vi "Instrumentation Controls.vi"() -> ()   [LabVIEW 2018]
doc: "This example shows how to use autosetup and acquire a waveform on a single channel."
uses:
  <instrlib>/RIGOL DG4000 Series/Public/Configure/Configure Standard Waveform(Sine).vi
  <instrlib>/RIGOL DS1000 Series/Public/Data/Read (Multiple Waveforms).vi
  <instrlib>/RIGOL DS1000 Series/RIGOL DS1000 Series.lvlib
  <instrlib>/RIGOL DM3058/RIGOL DM3058.lvlib
  <instrlib>/RIGOL DG4000 Series/RIGOL DG4000 Series.lvlib
panel:
  in  "Tab Control":enum32{"DG4062", "DM3068", "DS1204B"}(tab)
  in  "VISA resource name 2":refnum<visa-resource-name>
  in  "Amplitude (0.1 Vpp)":dbl=0.1
  in  "Frequency (1000 Hz)":dbl=1000.0
  in  "DC Offset (0.00 V)":dbl
  in  "Channel":dbl
  in  "Enable Output":bool=TRUE
  in  "VISA resource name 3":refnum<visa-resource-name>
  out "Measurement 3":dbl(knob) scale=0.0..5.0
  in  "Function (0: DC Volts) 2":u16(ring) items=["DC Volts", "AC Volts", "DC Current", "AC Current", "2-Wire Resistance", "4-Wire Resistance"]
  in  "Manual Range (1.0) 2":dbl=1.0
  in  "Auto Range (T: Enable) 2":bool=TRUE
  out "Measurement 4":dbl
  in  "VISA resource name":refnum<visa-resource-name>
  out "Waveform Data":waveform(dbl)[](graph)
  in  "Timeout (10000 ms)":u32=10000
  in  "Stop":bool
  in  "Channel (0: Channel 1)":u16[](array[ring]) items=["Channel 1", "Channel 2", "Channel 3", "Channel 4"]
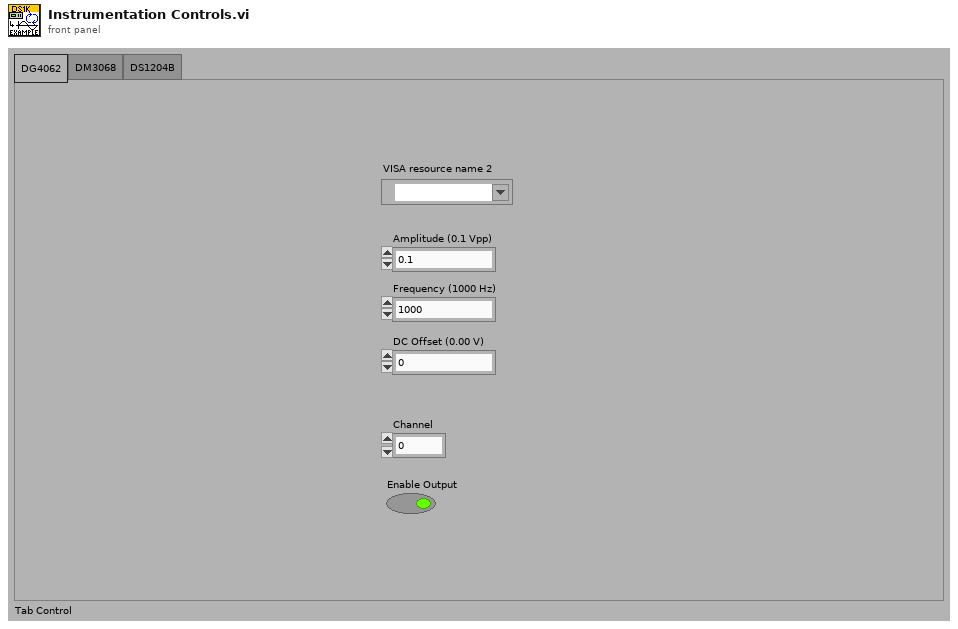
[diagram p1: front panel]
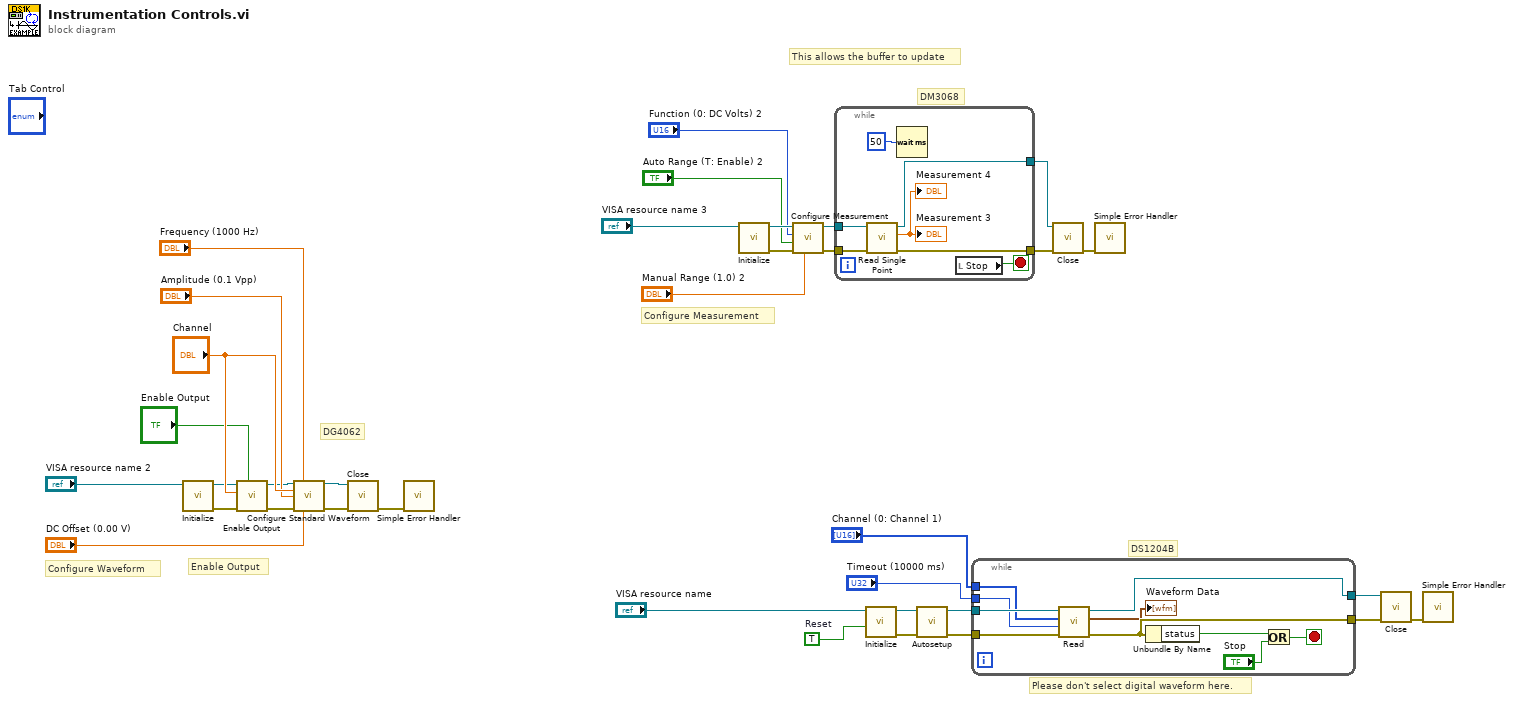
[diagram p0: block diagram]
diagram:
  w7 = TRUE  # Reset
  # "DG4062"
  # "DS1204B"
  # "This allows the buffer to update"
  # "Configure Measurement"
  # "Enable Output"
  # "Configure Waveform"
  # "DM3068"
  # "Please don't select digital waveform here."
  n1 = call <instrlib>:"Initialize.vi"("VISA resource name"="VISA resource name 2") -> ("error out"=w12:errorcluster, "VISA resource name out"=w11:refnum<visa-resource-name>)  [unwired: 4 in, 5 out]
  n2 = call <instrlib>:"Enable Output.vi"("Enable Output (T: Enable)"="Enable Output", "error in (no error)"=w12, "Output Channel (1: Channel 1)"="Channel", "VISA resource name"=w11) -> ("error out"=w14:errorcluster, "VISA resource name out"=w13:refnum<visa-resource-name>)  [unwired: 6 out]
  n3 = call-poly <instrlib>:"Configure Standard Waveform.vi"("VISA resource name"=w13, "Frequency (1000 Hz)"="Frequency (1000 Hz)", "Output Channel (1: Channel 1)"="Channel", "Amplitude (5 Vpp)"="Amplitude (0.1 Vpp)", "error in (no error)"=w14, "Offset (0)"="DC Offset (0.00 V)") -> ("VISA resource name out"=w18:refnum<visa-resource-name>, "error out"=w19:errorcluster)  [unwired: 8 in]
  n4 = call <instrlib>:"Close.vi"("error in (no error)"=w19, "VISA resource name"=w18) -> ("error out"=w8:errorcluster)  [unwired: 9 out]
  n5 = call <vilib>:"Simple Error Handler.vi"("error in (no error)"=w8) -> ()  [unwired: 1 in, 8 out]
  n6 = call <instrlib>:"Initialize.vi"("VISA resource name"="VISA resource name 3") -> ("error out"=w24:errorcluster, "VISA resource name out"=w25:refnum<visa-resource-name>)  [unwired: 4 in, 5 out]
  n7 = call <instrlib>:"Configure Measurement.vi"("Manual Range (1.00)"="Manual Range (1.0) 2", "error in (no error)"=w24, "Auto Range (T:Enable)"="Auto Range (T: Enable) 2", "Function (0: DC Volts)"="Function (0: DC Volts) 2", "VISA resource name"=w25) -> ("error out"=w4:errorcluster, "VISA resource name out"=w3:refnum<visa-resource-name>)  [unwired: 1 in, 4 out]
  n8 = while {
    tunnel: w3 -> [w42]
    tunnel: [w40] -> w31
    tunnel: w4 -> [w41]
    tunnel: [w39] -> w30
    stop <- w36 stop-if-true
    n9 = call <instrlib>:"Read Single Point.vi"("error in (no error)"=w41, "VISA resource name"=w42) -> ("error out"=w39:errorcluster, "Measurement"=→"Measurement 3" →"Measurement 4":dbl, "VISA resource name out"=w40:refnum<visa-resource-name>)  [unwired: 7 out]
    n10 = Wait (ms)(milliseconds to wait=u32 50) -> ()  [unwired: 1 out]
    n11 = local read "Stop"() -> (w36:bool)
  }
  n12 = call <instrlib>:"Initialize.vi"("Reset (True)"=w7, "VISA resource name"="VISA resource name") -> ("error out"=w28:errorcluster, "VISA resource name out"=w27:refnum<visa-resource-name>)  [unwired: 2 in, 6 out]
  n13 = call <instrlib>:"Autosetup.vi"("error in (no error)"=w28, "VISA resource name"=w27) -> ("error out"=w6:errorcluster, "VISA resource name out"=w5:refnum<visa-resource-name>)  [unwired: 8 out]
  n14 = while {
    tunnel: w5 -> [w52]
    tunnel: w6 -> [w51]
    tunnel: [w50] -> w34
    tunnel: [w48] -> w33
    tunnel: "Channel (0: Channel 1)" -> [w44]
    tunnel: "Timeout (10000 ms)" -> [w43]
    stop <- w49 stop-if-true
    n15 = call-poly <instrlib>:"Read.vi"("error in (no error)"=w51, "Timeout (10000 ms)"=w43, "Channels"=w44, "VISA resource name"=w52) -> ("error out"=w48:errorcluster, "Waveform Data"=→"Waveform Data":waveform(dbl)[], "VISA resource name out"=w50:refnum<visa-resource-name>)  [unwired: 5 out]
    n16 = Unbundle By Name(w48) -> ("status"=w47:bool)
    n17 = Or(x=w47, y="Stop") -> (x .or. y?=w49:bool)
  }
  n18 = call <instrlib>:"Close.vi"("error in (no error)"=w30, "VISA resource name"=w31) -> ("error out"=w32:errorcluster)  [unwired: 9 out]
  n19 = call <vilib>:"Simple Error Handler.vi"("error in (no error)"=w32) -> ()  [unwired: 1 in, 8 out]
  n20 = call <instrlib>:"Close.vi"("error in (no error)"=w33, "VISA resource name"=w34) -> ("error out"=w35:errorcluster)  [unwired: 9 out]
  n21 = call <vilib>:"Simple Error Handler.vi"("error in (no error)"=w35) -> ()  [unwired: 1 in, 8 out]
